vi "SlackAPI-oauth.v2.access.vi"(0 "code":string, 5 "client_id":string="1023330033985.1023512746241", 7 "client_secret":string="62f876b60829c507c6cb25bfe9dbba2b", 11 "error in (no error)":errorcluster) -> (4 "config":T1, 15 "error out":errorcluster)   [LabVIEW 2020]
uses:
  SlackAPI-oauth.v2.access response.ctl
  <vilib>/httpClient/POSTBuffer.vi
  <vilib>/httpClient/LabVIEWHTTPClient.lvlib
panel:
  out "body":string
  out "headers":string
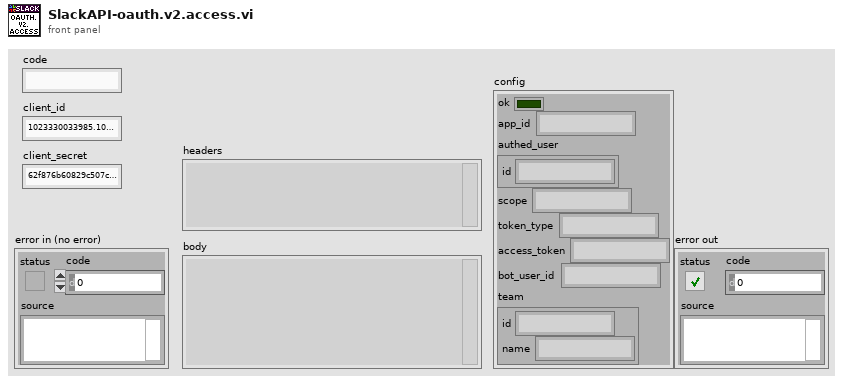
[diagram p1: front panel]
types:
  T1 = typedef "SlackAPI-oauth.v2.access response.ctl" = cluster{"ok":bool, "app_id":string, "authed_user":cluster{"id":string}, "scope":string, "token_type":string, "access_token":string, "bot_user_id":string, "team":cluster{"id":string, "name":string}}
  T2 = typedef "LabVIEWHTTPClient.lvlib/ClientHandle.ctl" = refnum<k1>
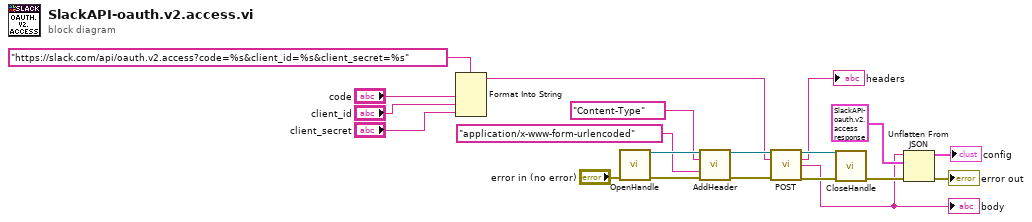
[diagram p0: block diagram]
diagram:
  n1 = Format Into String(format string="https://slack.com/api/oauth.v2.access?code=%s&client_id=%s&client_secret=%s", "code", "client_id", "client_secret") -> (resulting string=w12:string)  [unwired: 2 in, 1 out]
  n2 = call <vilib>:"OpenHandle.vi"("error in (no error)"="error in (no error)") -> ("client handle out"=w19:T2, "error out"=w20:errorcluster)  [unwired: 13 in]
  n3 = call <vilib>:"AddHeader.vi"("client handle"=w19, "header"="Content-Type", "value"="application/x-www-form-urlencoded", "error in (no error)"=w20) -> ("client handle out"=w15:T2, "error out"=w16:errorcluster)  [unwired: 10 in]
  n4 = call-poly <vilib>:"POST.vi"("client handle"=w15, "url"=w12, "error in (no error)"=w16) -> ("client handle out"=w11:T2, "headers"=→"headers":string, "body"=w2:string, "error out"=w10:errorcluster)  [unwired: 9 in]
  "body" <- w2
  n5 = call <vilib>:"CloseHandle.vi"("client handle"=w11, "error in (no error)"=w10) -> ("error out"=w6:errorcluster)  [unwired: 13 in]
  n6 = Unflatten From JSON(JSON string=w2, type and defaults=T1 {"ok"=TRUE, "app_id"="A010PF2MY73", "authed_user"={"id"="U010MS1SM43"}, "scope"="chat:write", "token_type"="bot", "access_token"="xoxb-1023330033985-1033540185744-vOlPQSl4eGew90iINuwHuUsW", "bot_user_id"="U010ZFW5FMW", "team"={"id"="T010P9Q0ZUZ", "name"="Development"}} ("Response"), error in (no error)=w6) -> (value=→"config":T1, error out=→"error out":errorcluster)  [unwired: 4 in]
